vi "温度PID控制.vi"() -> ()   [LabVIEW 2021]
uses:
  <vilib>/addons/control/pid/pid.llb/PID (DBL).vi
  <vilib>/addons/control/pid/NI_PID_pid.lvlib
panel:
  in  "停止":bool
  out "当前温度和设定温度":cluster{"initial PV":dbl, "SP:":dbl}(graph)
  in  "PID增益":T1={"比例增益(Kc)"=20.0, "积分时间（Ti，分）"=0.008, "微分时间（Td，分）"=0.001} {"微分时间（Td，分）" format="%.3f"; "积分时间（Ti，分）" format="%.3f"; "比例增益(Kc)" format="%.3f"}
  out "当前温度：":dbl(slide)=60.754431603254424 scale=0.0..100.0
  in  "设定温度：":dbl(slide)=43.790849673202615 min=0.0 max=0.0 scale=0.0..100.0
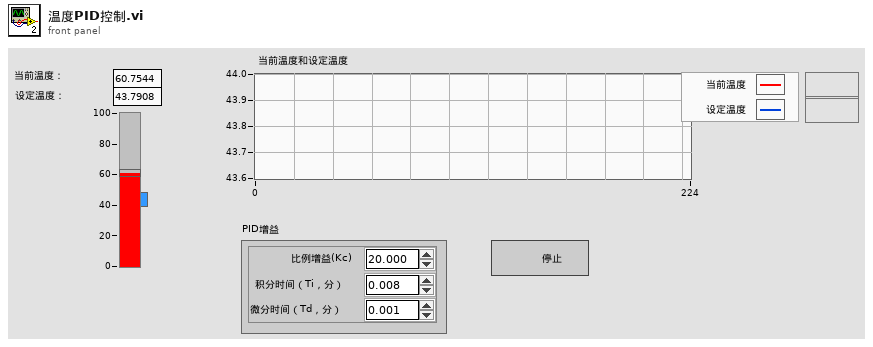
[diagram p1: front panel]
types:
  T1 = cluster{"比例增益(Kc)":dbl, "积分时间（Ti，分）":dbl, "微分时间（Td，分）":dbl}
  T2 = cluster{"static gain":dbl, "lag (min)":dbl, "dead cycles":dbl, "load %":dbl, "deadband":dbl, "noise level %":dbl, "initial PV":dbl, "initial PV 2":dbl}
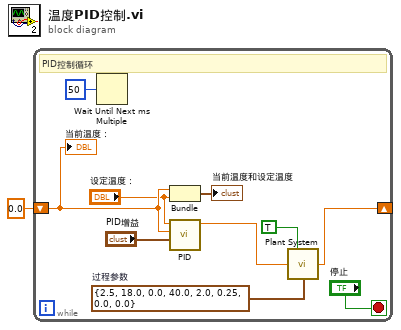
[diagram p0: block diagram]
diagram:
  n1 = while {
    shift-left: 0.0 ("设备输出") -> [w8]
    shift-right: [w10] -> _
    stop <- "停止" stop-if-true
    w3 = T2 {"static gain"=2.5, "lag (min)"=18.0, "dead cycles"=0.0, "load %"=40.0, "deadband"=2.0, "noise level %"=0.25, "initial PV"=0.0, "initial PV 2"=0.0}  # 过程参数
    # "PID控制循环"
    n2 = Wait Until Next ms Multiple(millisecond multiple=u32 50 ("unsigned 32bit integer")) -> ()  [unwired: 1 out]
    n3 = Bundle("设备输出"=w8, "设定温度："="设定温度：") -> (→"当前温度和设定温度":cluster{"设备输出":dbl, "设定温度：":dbl})  [unwired: 1 in]
    n4 = call-poly <vilib>:"PID.vi"("PID gains"="PID增益", "process variable"=w8, "setpoint"="设定温度：") -> ("output"=w4:dbl)  [unwired: 7 in, 1 out]
    n5 = call "Plant System.vi"("积分器？"=TRUE ("Integrator ?"), "设备输入"=w4, "过程参数"=w3) -> ("设备输出"=w10:dbl)  [unwired: 12 in]
    "当前温度：" <- w8
  }
